vi "Parse Parameter.vi"(6 "error text in":string, 8 "error in":errorcluster, 11 "node in":refnum<k20>) -> (0 "error out":errorcluster, 3 "parametesrs":T1[](array[typedef]) {"Parameter"."encoding" items=["BNR", "BCD", "Discrete", "Signed_32", "Signed_64", "Float_32", "Float_64", "Opaque"]})   [LabVIEW 2020, in "AIM ARINC 664 Import.lvlib"]
uses:
  AIM ARINC 664 Import.lvlib
  _typedefs/frame_parameter_definition.ctl
  _typedefs/frame_parameter.ctl
  Read Tag Element (String).vi
  Read Tag Element (DBL).vi
  Read Tag Element (I32).vi
  Read Tag Element (Boolean).vi
  Shared/Encoding (Arinc664).ctl
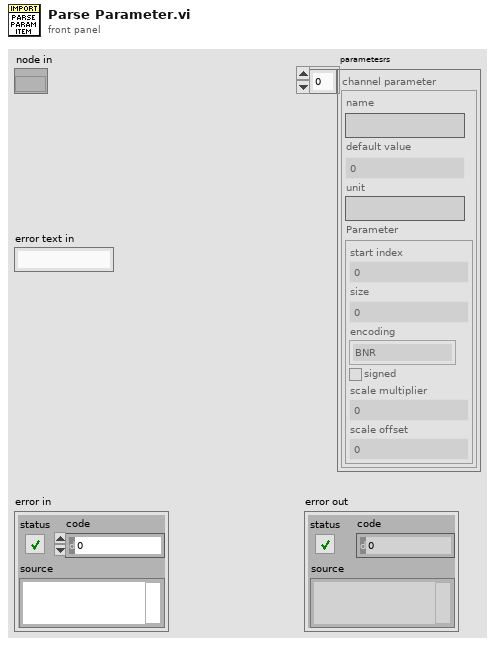
[diagram p1: front panel]
types:
  T1 = typedef "AIM ARINC 664 Import.lvlib/frame_parameter.ctl" = cluster{"name":string, "default value":dbl, "unit":string, "Parameter":T2}
  T2 = typedef "AIM ARINC 664 Import.lvlib/frame_parameter_definition.ctl" = cluster{"start index":i32, "size":i32, "encoding":T3, "signed":bool, "scale multiplier":dbl, "scale offset":dbl}
  T3 = typedef "Encoding (Arinc664).ctl" = u16
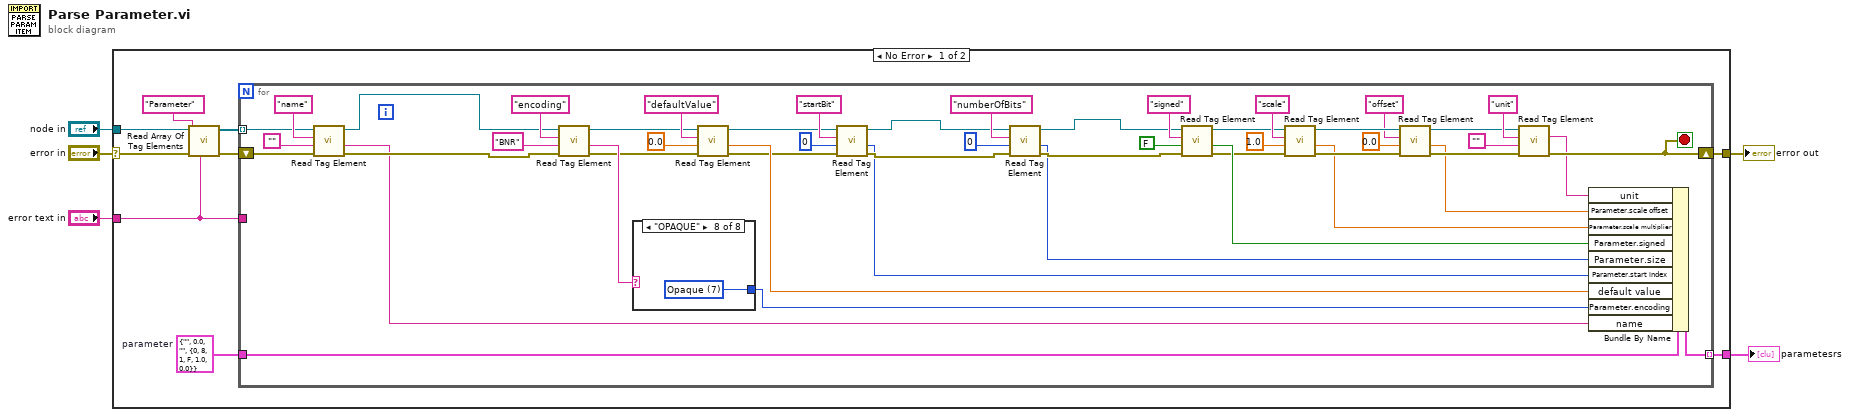
[diagram p0: block diagram]
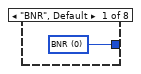
[diagram p2: hidden frame]
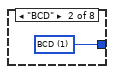
[diagram p3: hidden frame]
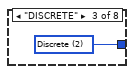
[diagram p4: hidden frame]
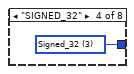
[diagram p5: hidden frame]
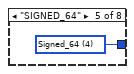
[diagram p6: hidden frame]
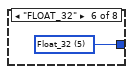
[diagram p7: hidden frame]
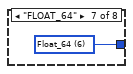
[diagram p8: hidden frame]
diagram:
  n1 = case shown="No Error" "error in" {
    selector: "error in" -> [w9 w72]
    tunnel: "node in" -> [w11 _]
    tunnel: [w10 w72] -> w4
    tunnel: "error text in" -> [w8 _]
    tunnel: [w7 _] -> w1
    frame No Error {
      w6 = T1 {"name"="", "default value"=0.0, "unit"="", "Parameter"={"start index"=0, "size"=8, "encoding"=1, "signed"=FALSE, "scale multiplier"=1.0, "scale offset"=0.0}}  # parameter
      n2 = call "Read Array Of Tag Elements.vi"("error text in"=w8, "error in"=w9, "tag name"="Parameter" ("Tag Name"), "node in"=w11) -> ("error out"=w13:errorcluster, "array of elements"=w12:refnum<k20>[])  [unwired: 6 in]
      n3 = for {
        shift-right: [w25] -> w10
        shift-left: w13 -> [w61]
        tunnel: w12 -> [w29] mode=indexing
        tunnel: w8 -> [_]
        tunnel: [w16] -> w7 mode=indexing
        tunnel: w6 -> [w15]
        stop <- w25 stop-if-true
        n4 = call-poly "Read Tag Element.vi"("error in"=w61, "default"="", "Tag Name"="name", "node in"=w29) -> ("error out"=w23:errorcluster, "value"=w20:string, "node out"=w22:refnum<k20>)  [unwired: 5 in]
        n5 = call-poly "Read Tag Element.vi"("error in"=w23, "default"="BNR", "Tag Name"="encoding", "node in"=w22) -> ("error out"=w54:errorcluster, "value"=w58:string, "node out"=w55:refnum<k20>)  [unwired: 5 in]
        n6 = case shown="\"OPAQUE\"" w58 {
          tunnel: [w64 w65 w66 w67 w68 w69 w70 w71] -> w21
          frame "BNR", Default {
            w64 = T3 0 items=["BNR", "BCD", "Discrete", "Signed_32", "Signed_64", "Float_32", "Float_64", "Opaque"] ("Encoding Type")
          }
          frame "BCD" {
            w65 = T3 1 items=["BNR", "BCD", "Discrete", "Signed_32", "Signed_64", "Float_32", "Float_64", "Opaque"] ("Encoding Type")
          }
          frame "DISCRETE" {
            w66 = T3 2 items=["BNR", "BCD", "Discrete", "Signed_32", "Signed_64", "Float_32", "Float_64", "Opaque"] ("Encoding Type")
          }
          frame "SIGNED_32" {
            w67 = T3 3 items=["BNR", "BCD", "Discrete", "Signed_32", "Signed_64", "Float_32", "Float_64", "Opaque"] ("Encoding Type")
          }
          frame "SIGNED_64" {
            w68 = T3 4 items=["BNR", "BCD", "Discrete", "Signed_32", "Signed_64", "Float_32", "Float_64", "Opaque"] ("Encoding Type")
          }
          frame "FLOAT_32" {
            w69 = T3 5 items=["BNR", "BCD", "Discrete", "Signed_32", "Signed_64", "Float_32", "Float_64", "Opaque"] ("Encoding Type")
          }
          frame "FLOAT_64" {
            w70 = T3 6 items=["BNR", "BCD", "Discrete", "Signed_32", "Signed_64", "Float_32", "Float_64", "Opaque"] ("Encoding Type")
          }
          frame "OPAQUE" {
            w71 = T3 7 items=["BNR", "BCD", "Discrete", "Signed_32", "Signed_64", "Float_32", "Float_64", "Opaque"] ("Encoding Type")
          }
        }
        n7 = call-poly "Read Tag Element.vi"("error in"=w54, "default"=0.0, "Tag Name"="defaultValue", "node in"=w55) -> ("error out"=w46:errorcluster, "value"=w53:dbl, "node out"=w50:refnum<k20>)  [unwired: 5 in]
        n8 = call-poly "Read Tag Element.vi"("error in"=w46, "default"=0, "Tag Name"="startBit", "node in"=w50) -> ("error out"=w28:errorcluster, "value"=w24:i32, "node out"=w47:refnum<k20>)  [unwired: 5 in]
        n9 = call-poly "Read Tag Element.vi"("error in"=w28, "default"=0, "Tag Name"="numberOfBits", "node in"=w47) -> ("error out"=w27:errorcluster, "value"=w26:i32, "node out"=w43:refnum<k20>)  [unwired: 5 in]
        n10 = call-poly "Read Tag Element.vi"("error in"=w27, "default"=FALSE, "Tag Name"="signed", "node in"=w43) -> ("error out"=w34:errorcluster, "value"=w42:bool, "node out"=w35:refnum<k20>)  [unwired: 5 in]
        n11 = call-poly "Read Tag Element.vi"("error in"=w34, "default"=1.0, "Tag Name"="scale", "node in"=w35) -> ("error out"=w41:errorcluster, "value"=w17:dbl, "node out"=w40:refnum<k20>)  [unwired: 5 in]
        n12 = call-poly "Read Tag Element.vi"("error in"=w41, "default"=0.0, "Tag Name"="offset", "node in"=w40) -> ("error out"=w30:errorcluster, "value"=w18:dbl, "node out"=w31:refnum<k20>)  [unwired: 5 in]
        n13 = call-poly "Read Tag Element.vi"("error in"=w30, "default"="", "Tag Name"="unit", "node in"=w31) -> ("error out"=w25:errorcluster, "value"=w19:string)  [unwired: 5 in, 1 out]
        n14 = Bundle By Name(cluster=w15, "unit"=w19, "Parameter.scale offset"=w18, "Parameter.scale multiplier"=w17, "Parameter.signed"=w42, "Parameter.size"=w26, "Parameter.start index"=w24, "default value"=w53, "Parameter.encoding"=w21, "name"=w20) -> (w16:T1)
      }
    }
    frame Error {
    }
  }
  "parametesrs" <- w1
  "error out" <- w4
